vi "LibreVNA Test 01.vi"() -> ()   [LabVIEW 2023]
uses:
  LibreVNA/Types/Trace Enum.ctl
  LibreVNA/LibreVNA.lvclass
  <userlib>/_OpenG.lib/time/time.llb/openg_time.lvlib
panel:
  out "Is Running":bool
  out "XY Graph":cluster{"Data Out":dbl[], "Data Out":dbl[]}(graph)
  in  "Trace Name":T1
  in  "Query Trace":bool
  in  "Query":bool
  in  "Command":string
  in  "SendCmd":bool
  in  "Stop":bool
  out "Recv Buffer":string
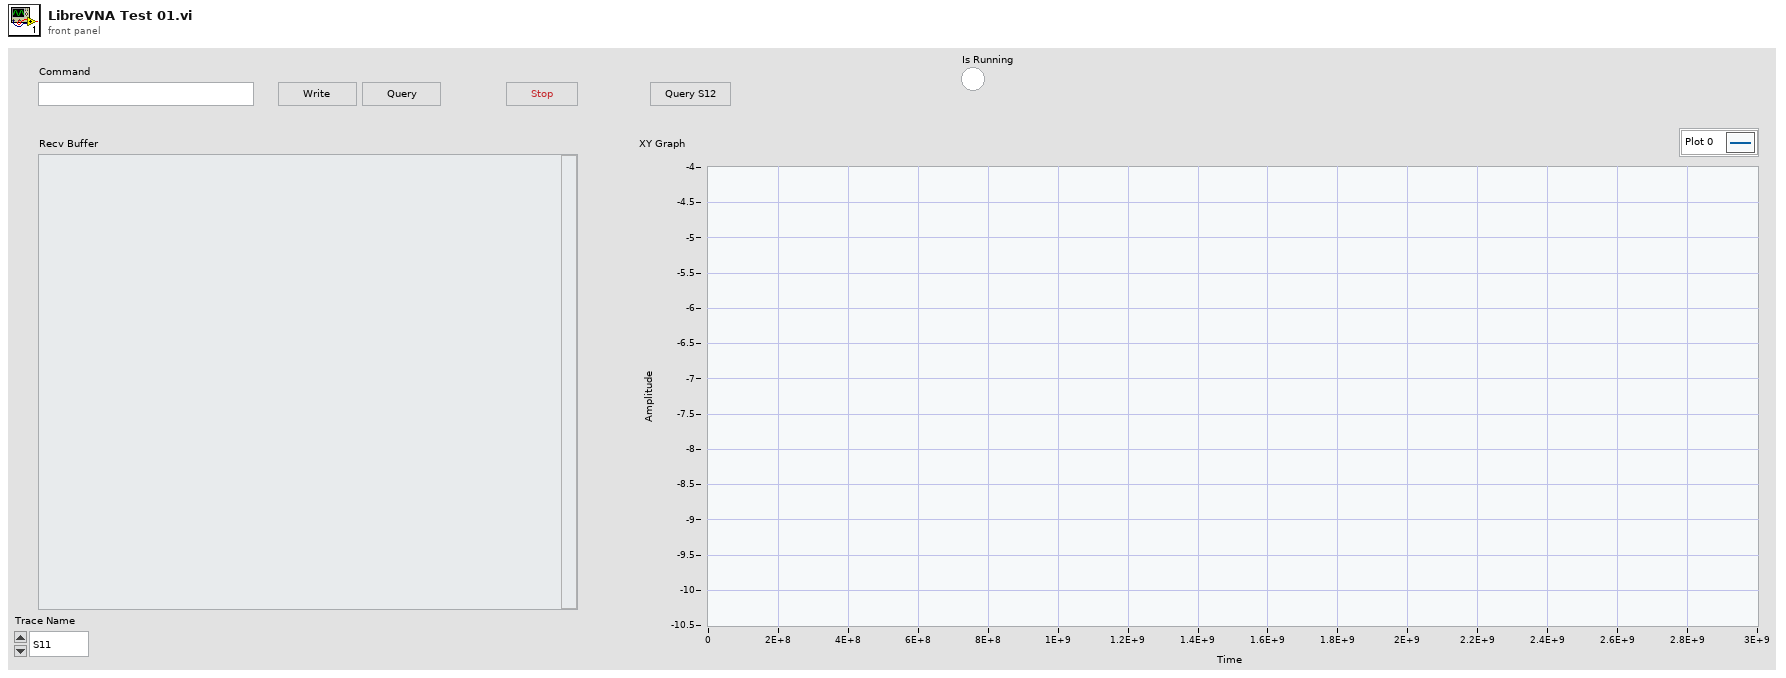
[diagram p1: front panel]
types:
  T1 = typedef "LibreVNA.lvclass/Trace Enum.ctl" = enum16{"S11", "S12", "S21", "S22"}
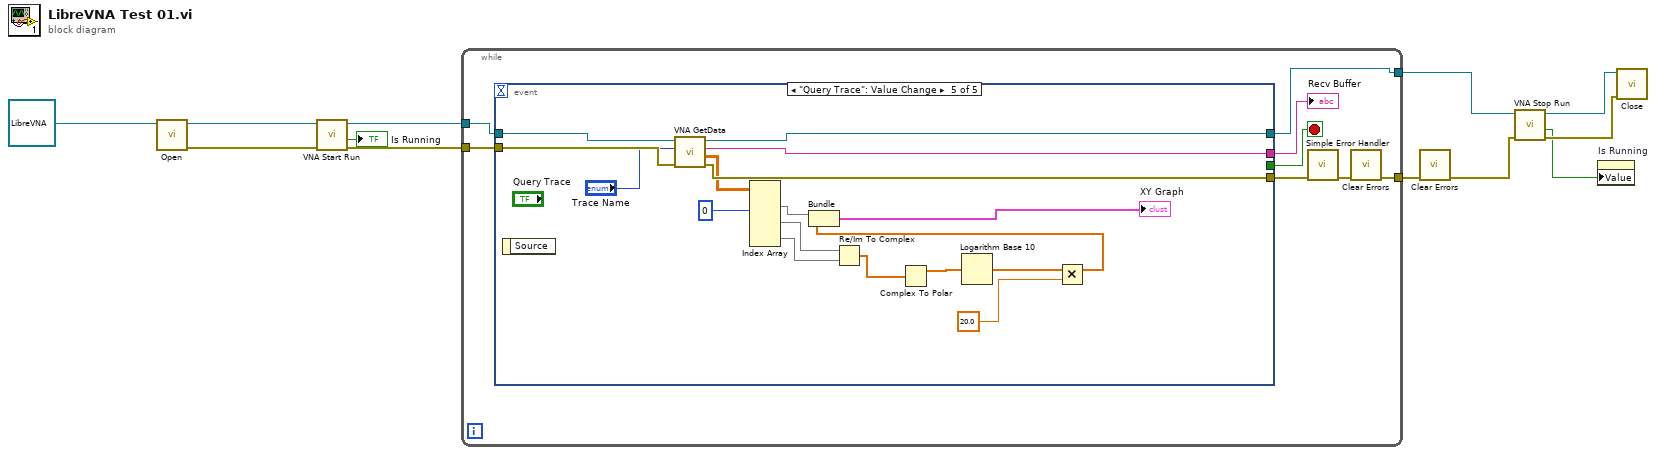
[diagram p0: block diagram]
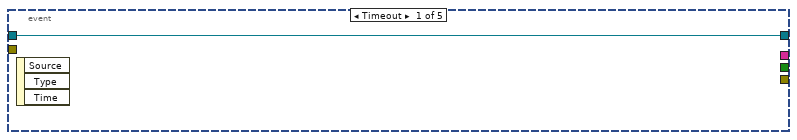
[diagram p2: hidden frame]
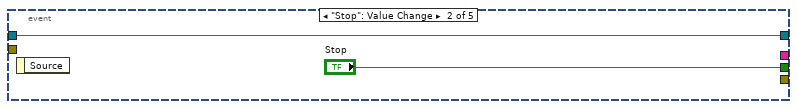
[diagram p3: hidden frame]
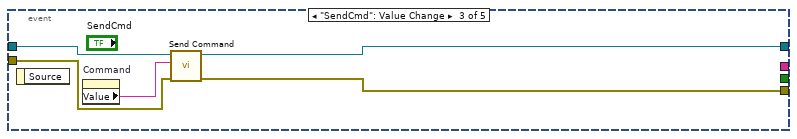
[diagram p4: hidden frame]
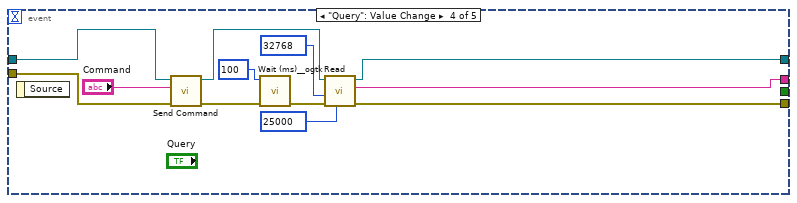
[diagram p5: hidden frame]
diagram:
  n1 = call-dynamic "Open.vi"("LibreVNA in"=refnum<class "LibreVNA.lvclass"> refnum ("LibreVNA.lvclass")) -> ("error out"=w8:errorcluster, "LibreVNA out"=w11:refnum<class "LibreVNA.lvclass">)  [unwired: 9 in]
  n2 = call-dynamic "VNA Start Run.vi"("error in (no error)"=w8, "LibreVNA in"=w11) -> ("error out"=w7:errorcluster, "Is Running"=→"Is Running":bool, "LibreVNA out"=w9:refnum<class "LibreVNA.lvclass">)  [unwired: 7 in]
  n3 = while {
    tunnel: w7 -> [w19]
    tunnel: w9 -> [w18]
    tunnel: [w14] -> w10
    tunnel: [w17] -> w6
    stop <- w20 stop-if-true
    n4 = event shown="[4] \"Query Trace\": Value Change" {
      selector: _ -> [_ _ _ _ _]
      dyn-events: _ -> [_ _ _ _ _]
      timeout: _ -> [_ _ _ _ _]
      tunnel: [_ "Stop" _ _ _] -> w20
      tunnel: w19 -> [_ _ w26 w32 w56]
      tunnel: w18 -> [w21 w22 w25 w33 w57]
      tunnel: [w21 w22 w27 w34 w54] -> w17
      tunnel: [_ _ w28 w31 w53] -> w15
      tunnel: [_ _ _ w30 w52] -> w13
      event Timeout {
        n5 = event-data() -> ()  [unwired: 1 in, 3 out]
      }
      event "Stop": Value Change {
        n6 = event-data() -> ()  [unwired: 1 in, 1 out]
      }
      event "SendCmd": Value Change {
        n7 = event-data() -> ()  [unwired: 1 in, 1 out]
        n8 = property on="Command" class="Str"() -> ("Value"=w24:string)  [unwired: 2 in, 2 out]
        n9 = call-dynamic "Send Command.vi"("error in (no error)"=w26, "Command"=w24, "LibreVNA in"=w25) -> ("error out"=w28:errorcluster, "LibreVNA out"=w27:refnum<class "LibreVNA.lvclass">)  [unwired: 6 in, 1 out]
      }
      event "Query": Value Change {
        n10 = event-data() -> ()  [unwired: 1 in, 1 out]
        n11 = call-dynamic "Send Command.vi"("error in (no error)"=w32, "Command"="Command", "LibreVNA in"=w33) -> ("error out"=w40:errorcluster, "LibreVNA out"=w39:refnum<class "LibreVNA.lvclass">)  [unwired: 6 in, 1 out]
        n12 = call <userlib>:"Wait (ms)__ogtk.vi"("error in (no error)"=w40, "milliseconds to wait"=u32 100) -> ("error out"=w37:errorcluster)  [unwired: 8 in, 1 out]
        n13 = call-dynamic "Read.vi"("timeout ms (5000)"=25000, "error in (no error)"=w37, "bytes to read"=32768, "LibreVNA in"=w39) -> ("error out"=w31:errorcluster, "Recv Buffer"=w30:string, "LibreVNA out"=w34:refnum<class "LibreVNA.lvclass">)  [unwired: 4 in, 1 out]
      }
      event "Query Trace": Value Change {
        n14 = event-data() -> ()  [unwired: 1 in, 1 out]
        n15 = call-dynamic "VNA GetData.vi"("error in (no error)"=w56, "Trace Name"="Trace Name", "LibreVNA in"=w57) -> ("error out"=w53:errorcluster, "Data Out"=w51:dbl[][], "Recv Buffer"=w52:string, "LibreVNA out"=w54:refnum<class "LibreVNA.lvclass">)  [unwired: 3 in, 2 out]
        n16 = Index Array(array=w51, index (col) #1=0 ("disabled index (col)")) -> (element #1=w49:dbl[], element #2=w47:dbl[], element #3=w46:dbl[])  [unwired: 5 in]
        n17 = Re/Im To Complex(1:w46, 2:w47) -> (0:w45:cdb[])
        n18 = Complex To Polar(r * e^(i*theta)=w45) -> (r=w44:dbl[])  [unwired: 1 out]
        n19 = Logarithm Base 10(1:w44) -> (0:w43:dbl[])
        n20 = Multiply(x=w43, y=20.0) -> (x*y=w42:dbl[])
        n21 = Bundle("Data Out"=w49, w42) -> (→"XY Graph":cluster{"Data Out":dbl[], dbl[]})  [unwired: 1 in]
      }
    }
    "Recv Buffer" <- w13
    n22 = call <vilib>:"Simple Error Handler.vi"("error in (no error)"=w15) -> ("error out"=w16:errorcluster)  [unwired: 4 in, 4 out]
    n23 = call <vilib>:"Clear Errors.vi"("error in (no error)"=w16) -> ("error out"=w14:errorcluster)  [unwired: 5 in, 1 out]
  }
  n24 = call <vilib>:"Clear Errors.vi"("error in (no error)"=w10) -> ("error out"=w4:errorcluster)  [unwired: 5 in, 1 out]
  n25 = call-dynamic "VNA Stop Run.vi"("error in (no error)"=w4, "LibreVNA in"=w6) -> ("error out"=w3:errorcluster, "Is Running"=w1:bool, "LibreVNA out"=w5:refnum<class "LibreVNA.lvclass">)  [unwired: 7 in]
  n26 = property on="Is Running" class="Bool (strict)"("Value"=w1) -> ()  [unwired: 2 in, 2 out]
  n27 = call-dynamic "Close.vi"("error in (no error)"=w3, "LibreVNA in"=w5) -> ()  [unwired: 8 in, 2 out]
